vi "main_o.vi"() -> ()   [LabVIEW 2016]
uses:
  Classes/Controller/Dispenser/Ultimus V2 Folder/Ultimus V2.lvclass
  Classes/Controller/Motion/Motion Folder/Motion.lvclass
  Classes/Controller/Motion/A3200 Folder/A3200.lvclass
  Classes/Controller/I-O/NI-DAQ Folder/NI-DAQ.lvclass
  D:/Gantry_General/Classes/Controller/Motion/Motion Folder/Motion.lvclass
  D:/Gantry_General/Classes/Controller/Controller Folder/Controller.lvclass
  D:/Gantry_General/Classes/Controller/Dispenser/Dispenser Folder/Dispenser.lvclass
  D:/Gantry_General/Classes/Controller/I-O/I-O Folder/I-O.lvclass
  Classes/Controller/I-O/I-O Folder/I-O.lvclass
  Classes/Controller/Dispenser/Dispenser Folder/Dispenser.lvclass
panel:
  out "XYZTheta Out":dbl[](array[numeric])
  in  "all control":T1={"controller"={"A3200.lvclass"=refnum, "Ultimus V2.lvclass"=refnum, "NI-DAQ.lvclass"=refnum}, "IO"={"Output num"=[], "Output "=[]}, "motion"={"XYZU "=[], "speed"=0.0}, "dispense"={"Vacuum Setting (0000)"=0, "Pressure"=20, "on delay (ms)"=0.5, "off delay (ms) "=0.5}, "folder and file name"={"Path"=path "D:/Gantry_General/Main/ms_kao", "folder name"="data", "file name"="data_", "extension"="txt", "add time string"=FALSE}} {"dispense"."Vacuum Setting (0000)" min=0 max=1000 step=1 format="%04.0f"}
  in  "Tab Control":enum32{"dispenser", "motion", "IO", "file"}(tab)
  in  "dispense":T2={"Vacuum Setting (0000)"=0, "Pressure"=20, "on delay (ms)"=0.5, "off delay (ms) "=0.5} {"Vacuum Setting (0000)" min=0 max=1000 step=1 format="%04.0f"}
  in  "dispense change status":bool
  in  "Position":dbl format="%#_13g"
  in  "Z Go":bool
  in  "Z move to zero":bool
  in  "motion":cluster{"XYZU ":dbl[], "speed":dbl}
  in  "XY":dbl[](array[numeric])
  in  "XY Go":bool
  in  "joystick":bool
  out "Output":bool[](array[boolean])
  in  "IO":cluster{"Output num":dbl[], "Output ":bool[]}
  in  "folder and file name":T3={"Path"=path "D:/Gantry_General/Main/ms_kao", "folder name"="data", "file name"="data_", "extension"="txt", "add time string"=FALSE}
  in  "joystick and camera":bool
  in  "move to center":bool
  in  "move to needle position":bool
  in  "stop":bool
  in  "go":bool
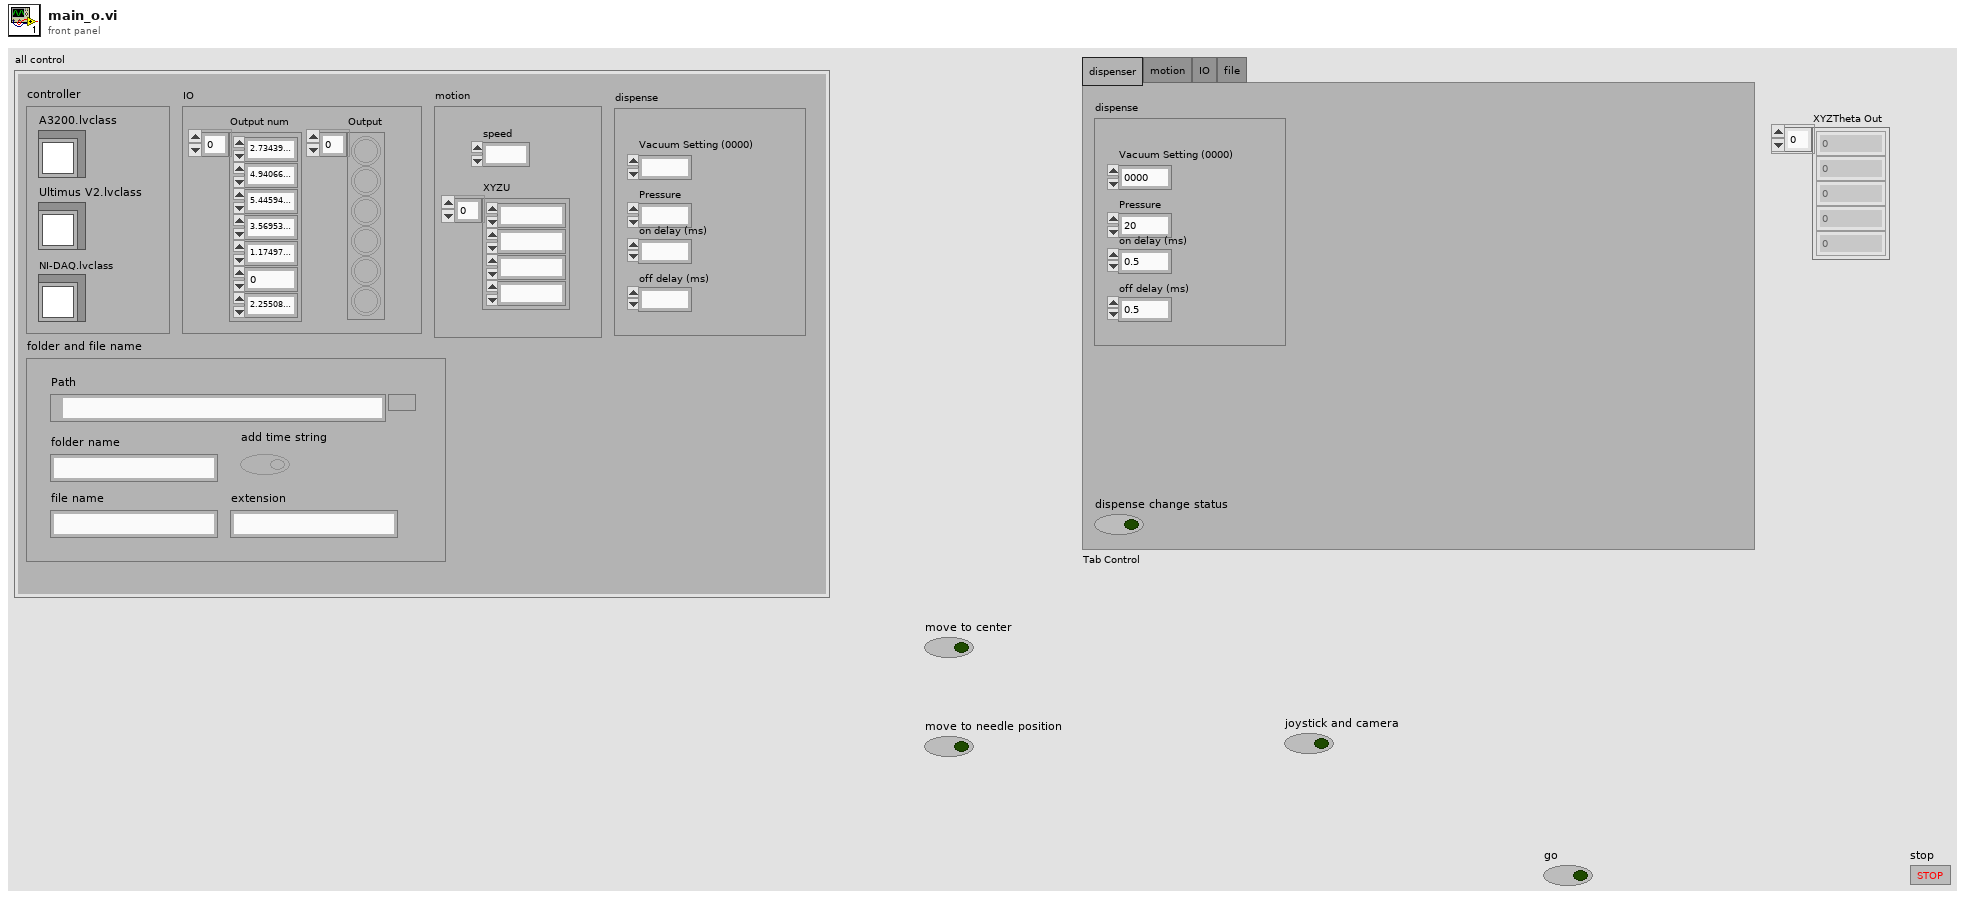
[diagram p1: front panel]
types:
  T1 = cluster{"controller":cluster{"A3200.lvclass":refnum<class "A3200.lvclass">, "Ultimus V2.lvclass":refnum<class "Ultimus V2.lvclass">, "NI-DAQ.lvclass":refnum<class "NI-DAQ.lvclass">}, "IO":cluster{"Output num":dbl[], "Output ":bool[]}, "motion":cluster{"XYZU ":dbl[], "speed":dbl}, "dispense":cluster{"Vacuum Setting (0000)":i64, "Pressure":i16, "on delay (ms)":dbl, "off delay (ms) ":dbl}, "folder and file name":cluster{"Path":path, "folder name":string, "file name":string, "extension":string, "add time string":bool}}
  T2 = cluster{"Vacuum Setting (0000)":i64, "Pressure":i16, "on delay (ms)":dbl, "off delay (ms) ":dbl}
  T3 = cluster{"Path":path, "folder name":string, "file name":string, "extension":string, "add time string":bool}
  T4 = cluster{"A3200.lvclass":refnum<class "A3200.lvclass">, "Ultimus V2.lvclass":refnum<class "Ultimus V2.lvclass">, "NI-DAQ.lvclass":refnum<class "NI-DAQ.lvclass">}
  T5 = cluster{"A3200.lvclass":refnum<class "A3200.lvclass">, "Ultimus V2.lvclass":refnum<class "Ultimus V2.lvclass">, "NI-DAQ.lvclass":refnum<class "NI-DAQ.lvclass">, "Motion.lvclass":refnum<class "Motion.lvclass">, "I-O.lvclass":refnum<class "I-O.lvclass">, "Dispenser.lvclass":refnum<class "Dispenser.lvclass">}
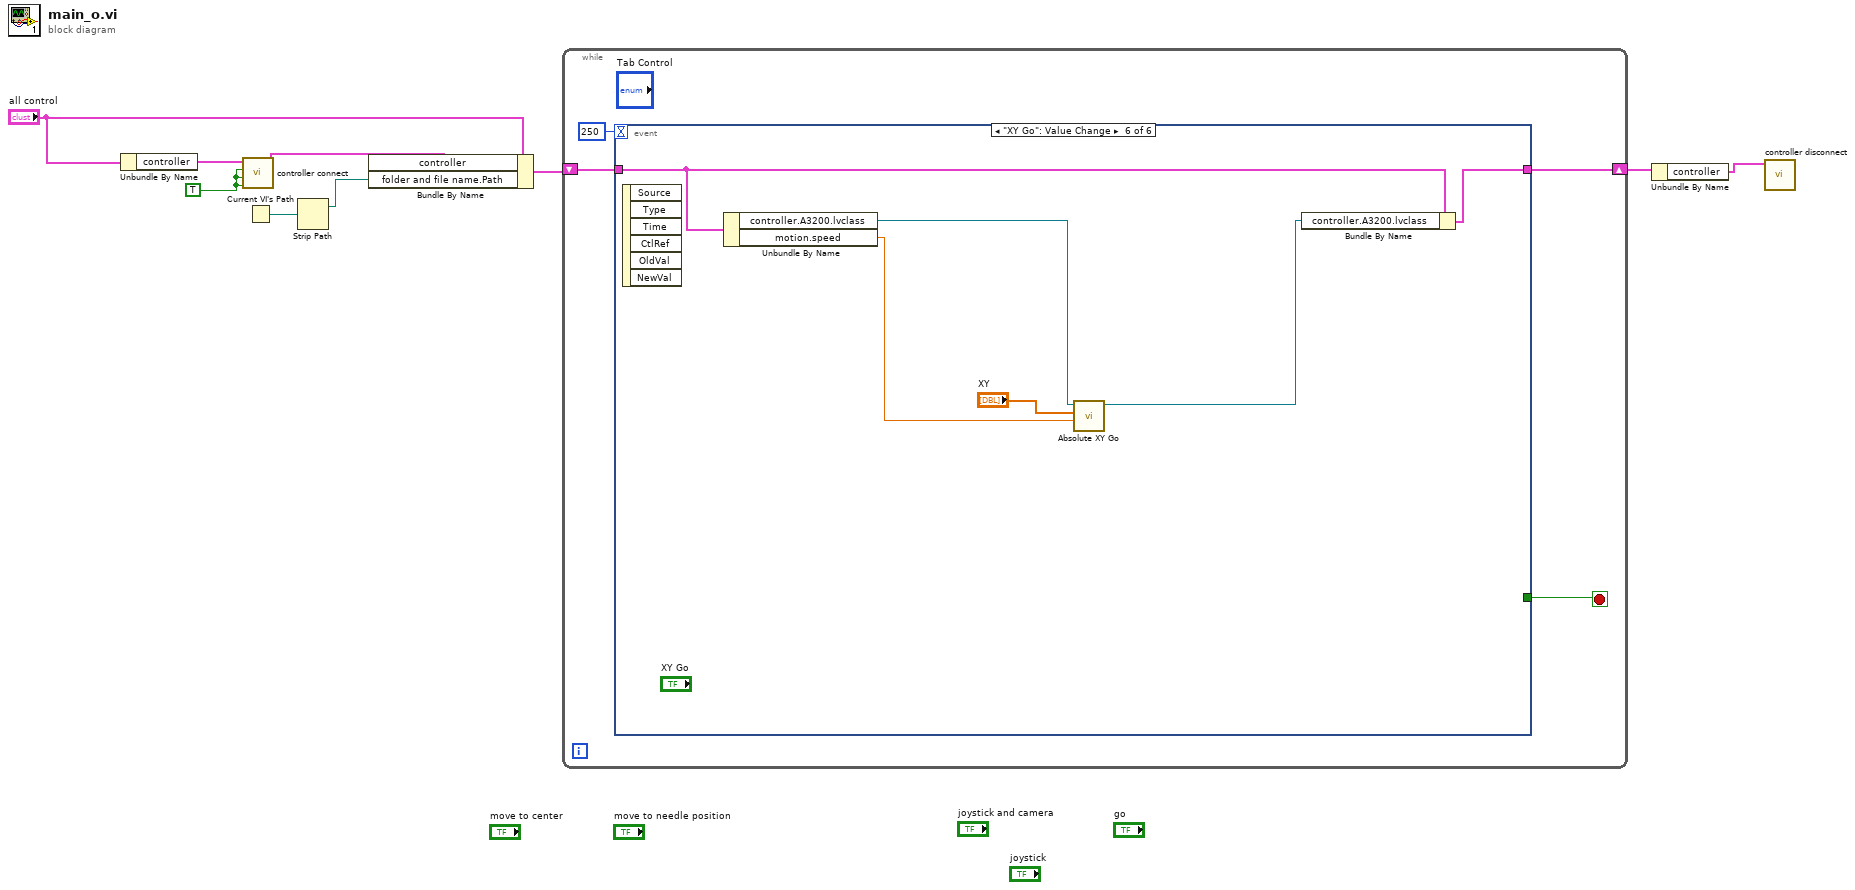
[diagram p0: block diagram]
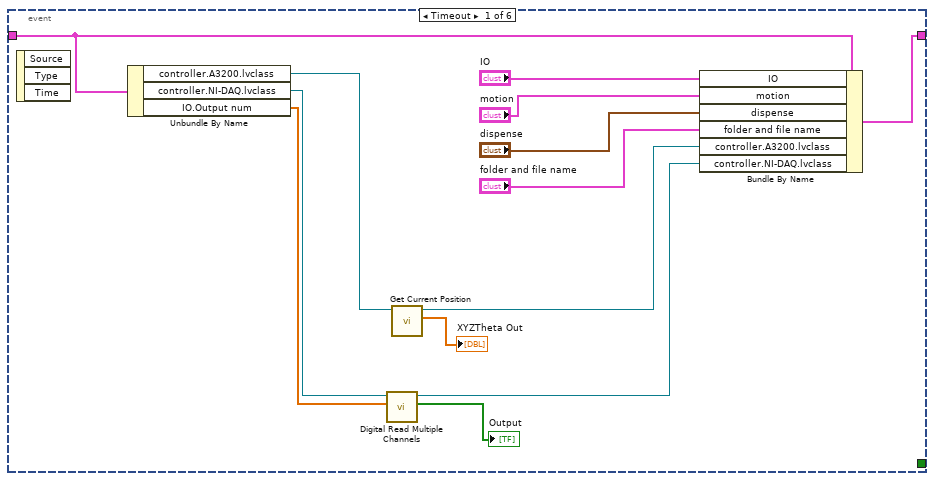
[diagram p2: hidden frame]
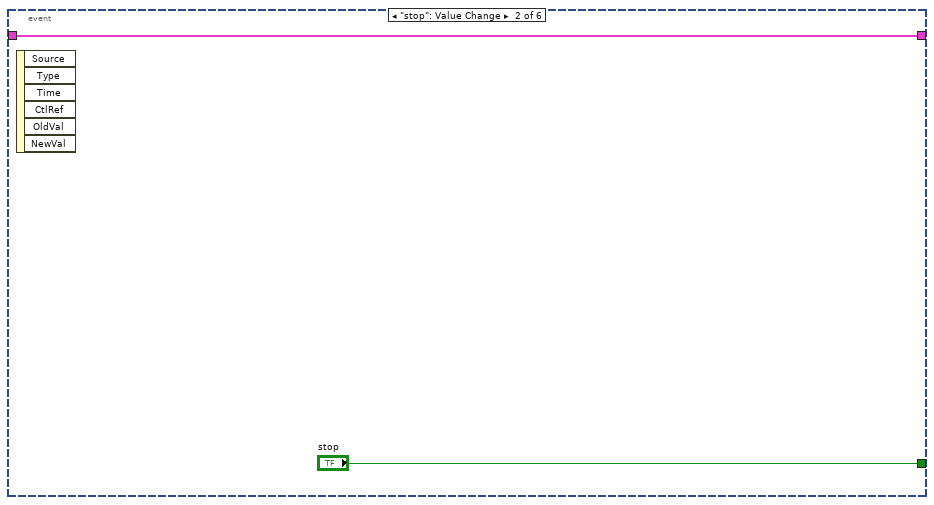
[diagram p3: hidden frame]
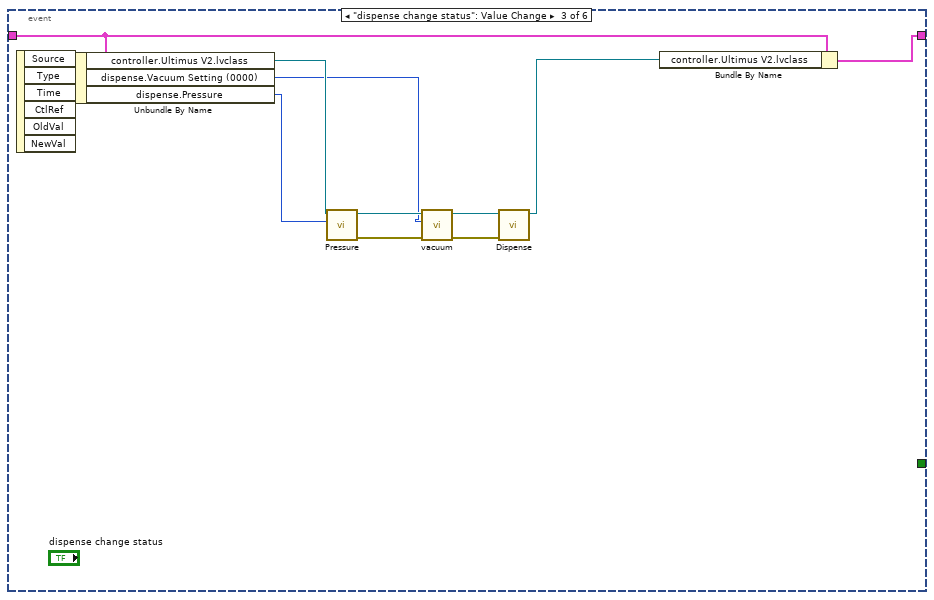
[diagram p4: hidden frame]
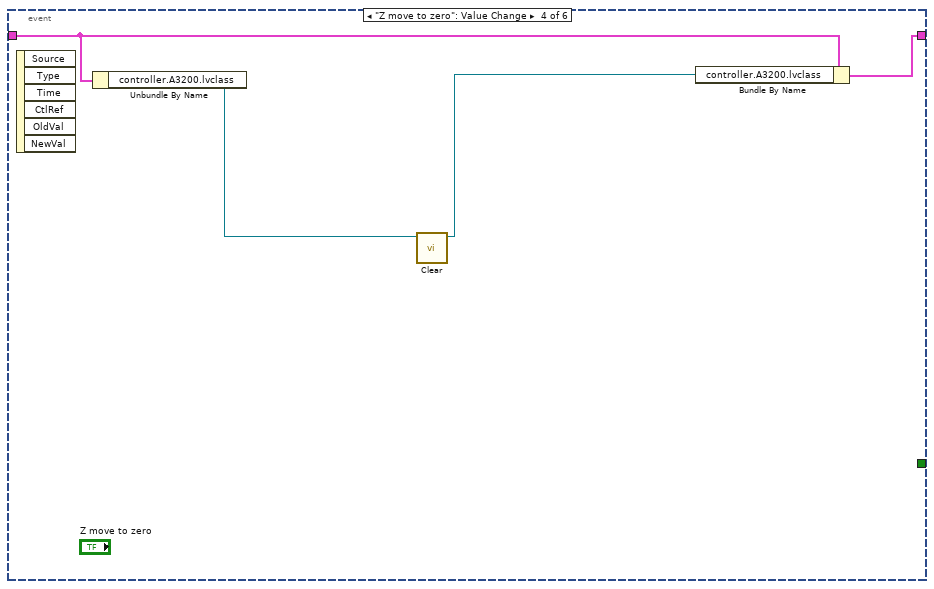
[diagram p5: hidden frame]
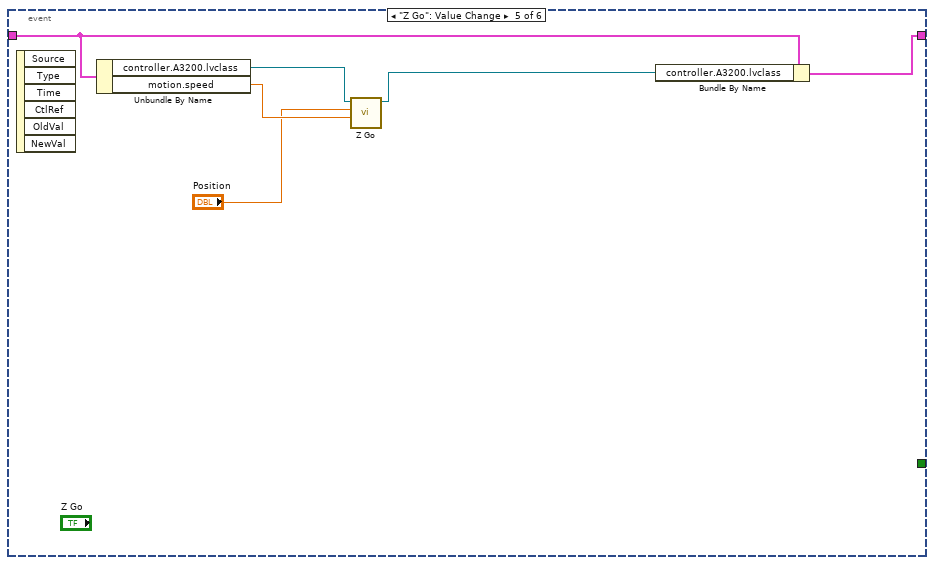
[diagram p6: hidden frame]
diagram:
  w9 = TRUE
  n1 = Unbundle By Name("all control") -> ("controller"=w8:T4)
  n2 = call "controller connect.vi"("IO on"=w9, "dispencer on"=w9, "motion on"=w9, "controller in"=w8) -> ("controller out"=w6:T5)  [unwired: 7 in]
  n3 = Current VI's Path() -> (path=w3:path)
  n4 = Strip Path(path=w3) -> (stripped path=w4:path)  [unwired: 1 out]
  n5 = Bundle By Name(cluster="all control", "controller"=w6, "folder and file name.Path"=w4) -> (w5:T1)
  n6 = while {
    shift-right: [w10] -> w2
    shift-left: w5 -> [w11]
    stop <- w13 stop-if-true
    n7 = event shown="[5] \"XY Go\": Value Change" {
      selector: _ -> [_ _ _ _ _ _]
      dyn-events: _ -> [_ _ _ _ _ _]
      timeout: 250 -> [_ _ _ _ _ _]
      tunnel: [_ "stop" _ _ _ _] -> w13
      tunnel: w11 -> [w26 w27 w37 w41 w48 w54]
      tunnel: [w25 w27 w38 w42 w45 w53] -> w10
      event Timeout {
        n8 = event-data() -> ()  [unwired: 1 in, 3 out]
        n9 = Unbundle By Name(w26) -> ("controller.A3200.lvclass"=w20:refnum<class "A3200.lvclass">, "controller.NI-DAQ.lvclass"=w19:refnum<class "NI-DAQ.lvclass">, "IO.Output num"=w18:dbl[])
        n10 = call-dynamic "Digital Read Multiple Channels.vi"("Array"=w18, "NI-DAQ in"=w19) -> ("subarray"=→"Output":bool[], "NI-DAQ out"=w16:refnum<class "NI-DAQ.lvclass">)  [unwired: 7 in, 1 out]
        n11 = call-dynamic "Get Current Position.vi"("Gantry in"=w20) -> ("XYZTheta Out"=→"XYZTheta Out":dbl[], "Gantry out"=w17:refnum<class "A3200.lvclass">)  [unwired: 8 in, 1 out]
        n12 = Bundle By Name(cluster=w26, "IO"="IO", "motion"="motion", "dispense"="dispense", "folder and file name"="folder and file name", "controller.A3200.lvclass"=w17, "controller.NI-DAQ.lvclass"=w16) -> (w25:T1)
      }
      event "stop": Value Change {
        n13 = event-data() -> ()  [unwired: 1 in, 6 out]
      }
      event "dispense change status": Value Change {
        n14 = event-data() -> ()  [unwired: 1 in, 6 out]
        n15 = Unbundle By Name(w37) -> ("controller.Ultimus V2.lvclass"=w36:refnum<class "Ultimus V2.lvclass">, "dispense.Vacuum Setting (0000)"=w29:i64, "dispense.Pressure"=w30:i16)
        n16 = call-dynamic "Pressure.vi"("Pressure"=w30, "Ultimus V in"=w36) -> ("error out"=w32:errorcluster, "Ultimus V out"=w35:refnum<class "Ultimus V2.lvclass">)  [unwired: 8 in]
        n17 = call "vacuum.vi"("error in (no error)"=w32, "Vacuum Setting (0000)"=w29, "Ultimus V in"=w35) -> ("error out"=w31:errorcluster, "Ultimus V out"=w34:refnum<class "Ultimus V2.lvclass">)  [unwired: 7 in]
        n18 = call-dynamic "Dispense.vi"("error in (no error)"=w31, "Ultimus V in"=w34) -> ("Ultimus V out"=w33:refnum<class "Ultimus V2.lvclass">)  [unwired: 8 in, 1 out]
        n19 = Bundle By Name(cluster=w37, "controller.Ultimus V2.lvclass"=w33) -> (w38:T1)
      }
      event "Z move to zero": Value Change {
        n20 = event-data() -> ()  [unwired: 1 in, 6 out]
        n21 = Unbundle By Name(w41) -> ("controller.A3200.lvclass"=w40:refnum<class "A3200.lvclass">)
        n22 = call "Clear.vi"("Motion in"=w40) -> ("Motion out"=w39:refnum<class "A3200.lvclass">)  [unwired: 9 in, 1 out]
        n23 = Bundle By Name(cluster=w41, "controller.A3200.lvclass"=w39) -> (w42:T1)
      }
      event "Z Go": Value Change {
        n24 = event-data() -> ()  [unwired: 1 in, 6 out]
        n25 = Unbundle By Name(w48) -> ("controller.A3200.lvclass"=w47:refnum<class "A3200.lvclass">, "motion.speed"=w44:dbl)
        n26 = call-dynamic "Z Go.vi"("Speed"=w44, "Position"="Position", "Gantry in"=w47) -> ("Gantry out"=w46:refnum<class "A3200.lvclass">)  [unwired: 7 in, 1 out]
        n27 = Bundle By Name(cluster=w48, "controller.A3200.lvclass"=w46) -> (w45:T1)
      }
      event "XY Go": Value Change {
        n28 = event-data() -> ()  [unwired: 1 in, 6 out]
        n29 = Unbundle By Name(w54) -> ("controller.A3200.lvclass"=w51:refnum<class "A3200.lvclass">, "motion.speed"=w50:dbl)
        n30 = call-dynamic "Absolute XY Go.vi"("Speed"=w50, "XY"="XY", "Gantry in"=w51) -> ("Gantry out"=w52:refnum<class "A3200.lvclass">)  [unwired: 7 in, 1 out]
        n31 = Bundle By Name(cluster=w54, "controller.A3200.lvclass"=w52) -> (w53:T1)
      }
    }
  }
  n32 = Unbundle By Name(w2) -> ("controller"=w1:T4)
  n33 = call "controller disconnect.vi"("controller 2"=w1) -> ()  [unwired: 11 in]
